vi "WPI_IMU_Loop.vi"(8 "error in":errorcluster, 11 "ADI IMU Interrupt DevRef":T1={"SimpleGyroDevRef"={"DevStatus"={"status"=FALSE, "code"=0, "source"=""}, "Handle"=0, "SPI Bus"=enum."SPI On-Board, CS0", "Device Found"=FALSE, "Sample Rate"=0.0, "Device Ready"=FALSE, "Yaw Axis"=enum."Z", "AHRS Algorithm"=enum."Complementary"}, "InterruptRef"={"DevStatus"={"status"=FALSE, "code"=0, "source"=""}, "InterruptIndex"=enum."0"}} {"SimpleGyroDevRef"."Sample Rate" min=0.25 max=100.0 step=0.25}) -> (0 "error out":errorcluster, 1 "Device Found":bool)   [LabVIEW 2015, in "FRC ADI MXP IMU.lvlib"]
doc: "Periodically reads the ADI MXP IMU valuse and makes data available for use elsewhere in your robot project. Place this block within PeriodicTasks.vi outside any loops."
uses:
  FRC ADI MXP IMU.lvlib
  WPI_AnalogDevicesIMUInterruptDevRef.ctl
  WPI_AnalogDevicesIMUDevRef.ctl
  <vilib>/Rock Robotics/SystemInterfaces/spilib/spi_bus.ctl
  <vilib>/Rock Robotics/WPI/Interrupt/WPI_InterruptRef.ctl
  <vilib>/Rock Robotics/SystemInterfaces/Interrupt/FPGA_InterruptIndex.ctl
  <vilib>/Rock Robotics/WPI/SPI/WPI_SPIDevRef.ctl
  <vilib>/Platform/TimedLoop/XDataNode/timing_clust.ctl
  <vilib>/Platform/TimedLoop/XDataNode/nitl_modes.ctl
  <vilib>/Platform/TimedLoop/XDataNode/wakeup.ctl
  <vilib>/Rock Robotics/SystemInterfaces/Interrupt/FPGA_WaitOnInterrupt.vi
  <vilib>/Rock Robotics/WPI/Utilities/WPI_UtilitiesTimebaseConstants.vi
  <vilib>/Rock Robotics/SystemInterfaces/Interrupt/FPGA_InterruptReadTimestamp.vi
  <vilib>/platform/TimedLoop/XDataNode/XDataNode.xnode
  <vilib>/ptbypt/NI_PtbyPt.lvlib
  <vilib>/Platform/TimedLoop/XDataNode/XDNodeRunTimeDep.lvlib
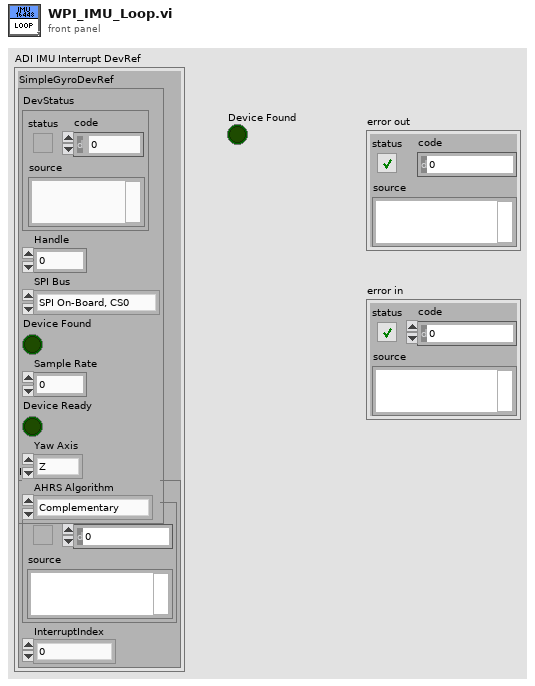
[diagram p1: front panel]
types:
  T1 = typedef "FRC ADI MXP IMU.lvlib/WPI_AnalogDevicesIMUInterruptDevRef.ctl" = cluster{"SimpleGyroDevRef":T2, "InterruptRef":T4}
  T2 = typedef "FRC ADI MXP IMU.lvlib/WPI_AnalogDevicesIMUDevRef.ctl" = cluster{"DevStatus":errorcluster, "Handle":i32, "SPI Bus":T3, "Device Found":bool, "Sample Rate":dbl, "Device Ready":bool, "Yaw Axis":enum16{"X", "Y", "Z"}, "AHRS Algorithm":enum16{"Complementary", "Madgwick"}}
  T3 = typedef "spi_bus.ctl" = enum16{"SPI On-Board, CS0", "SPI On-Board, CS1", "SPI On-Board, CS2", "SPI On-Board, CS3", "SPI MXP", "Invalid"}
  T4 = typedef "WPI_InterruptRef.ctl" = cluster{"DevStatus":errorcluster, "InterruptIndex":T5}
  T5 = typedef "FPGA_InterruptIndex.ctl" = enum8{"0", "1", "2", "3", "4", "5", "6", "7", "Invalid"}
  T6 = typedef "WPI_SPIDevRef.ctl" = cluster{"DevStatus":errorcluster, "Handle":i32, "SPI Bus":T3}
  T7 = cluster{"X Crossover":dbl, "Y Crossover":dbl, "Z Crossover":dbl, "X Range":dbl, "Y Range":dbl, "Z Range":dbl, "X Angle":dbl, "Y Angle":dbl, "Z Angle":dbl}
  T8 = cluster{"Output[0]":dbl, "Output[1]":dbl, "Output[2]":dbl}
  T9 = typedef "XDNodeRunTimeDep.lvlib/timing_clust.ctl" = cluster{"Expected End [f-1]":u64, "Actual End [f-1]":u64, "Finished Late? [f-1]":bool, "Expected End [i-1]":u64, "Actual End [i-1]":u64, "Finished Late? [i-1]":bool, "Expected Start [i]":u64, "Actual Start [i]":u64, "Expected Start [f]":u64, "Actual Start [f]":u64, "Source Name":string, "Structure Name":string, "Period":i64, "Deadline":i64, "Offset":i64, "Start":i64, "Priority":i32, "Timeout":i32, "Mode":T10, "Wakeup Reason":T11, "Error":errorcluster, "Source Type":string, "Secondary Source Type":string, "Global End Time":u64, "Global Start Time":u64, "Frame Duration":u64, "Iteration Duration":u64, "Assigned CPU":i32, "I/O Scan Engine Mode":u32}
  T10 = typedef "XDNodeRunTimeDep.lvlib/nitl_modes.ctl" = enum32{"No Change", "Process missed periods, maintain original phase", "Discard missed periods, maintain original phase", "Process missed periods, ignore original phase", "Discard missed periods, ignore original phase"}
  T11 = typedef "XDNodeRunTimeDep.lvlib/wakeup.ctl" = enum32{"Normal", "Aborted", "Asynchronous wakeup", "Timing source error", "Timed loop error", "Timeout"}
  T12 = cluster{"Data Array[0]":dbl, "Data Array[1]":dbl, "Data Array[2]":dbl, "Data Array[3]":dbl, "Data Array[4]":dbl, "Data Array[5]":dbl, "Data Array[6]":dbl, "Data Array[7]":dbl, "Data Array[8]":dbl, "Data Array[9]":dbl, "Data Array[10]":dbl}
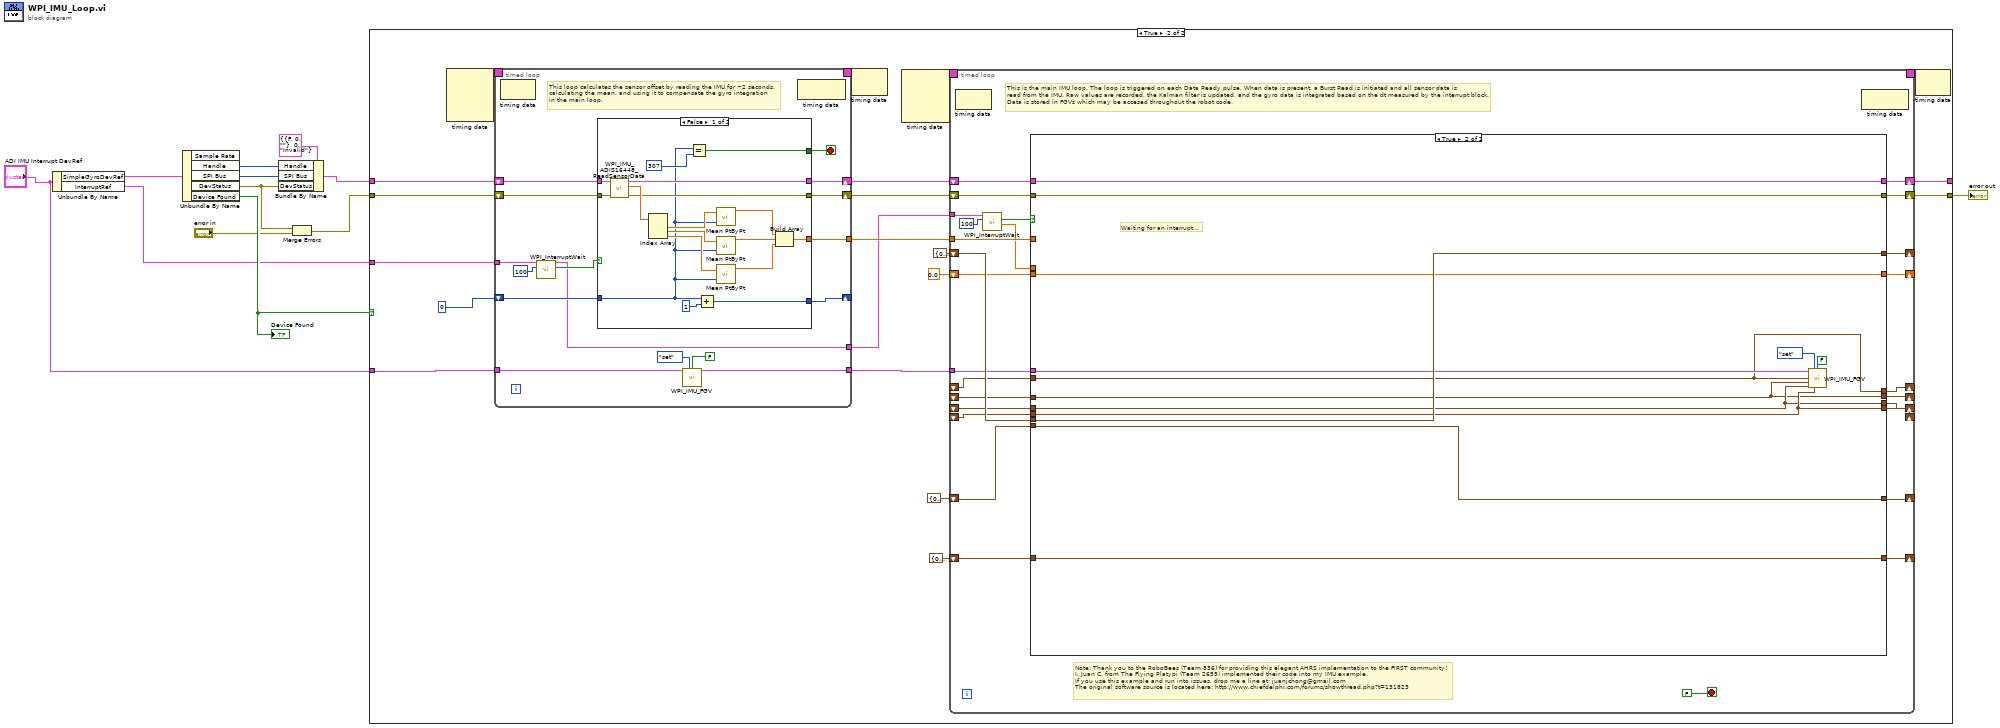
[diagram p0: block diagram]
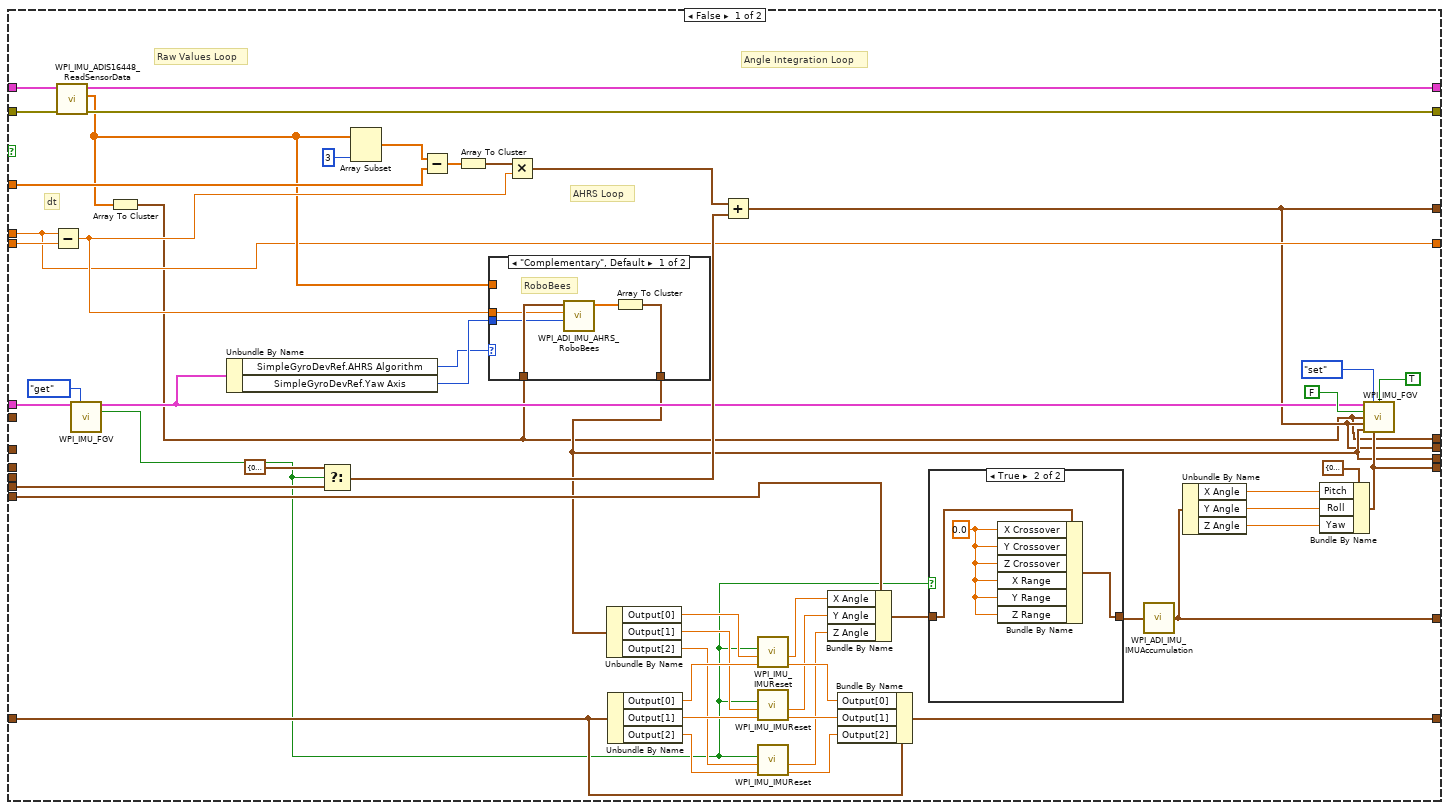
[diagram p3: hidden frame]
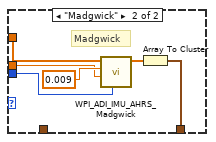
[diagram p5: hidden frame]
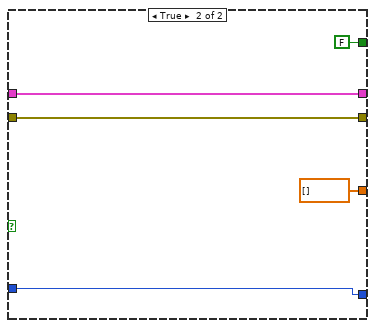
[diagram p6: hidden frame]
diagram:
  n1 = Unbundle By Name("ADI IMU Interrupt DevRef") -> ("SimpleGyroDevRef"=w6:T2, "InterruptRef"=w5:T4)
  n2 = Unbundle By Name(w6) -> ("Handle"=w11:i32, "SPI Bus"=w10:T3, "DevStatus"=w3:errorcluster, "Device Found"=w9:bool)  [unwired: 1 out]
  "Device Found" <- w9
  n3 = Bundle By Name(cluster=T6 {"DevStatus"={"status"=FALSE, "code"=0, "source"=""}, "Handle"=0, "SPI Bus"=enum."Invalid"} ("SPIDevRef out"), "Handle"=w11, "SPI Bus"=w10, "DevStatus"=w3) -> (w8:T6)
  n4 = Merge Errors(w3, "error in") -> (w1:errorcluster)
  n5 = case shown="True" w9 {
    tunnel: w8 -> [w14 w32]
    tunnel: w1 -> [w13 w31]
    tunnel: [w13 w34] -> w7
    tunnel: [w14 w33] -> _
    tunnel: "ADI IMU Interrupt DevRef" -> [_ w19]
    tunnel: w5 -> [_ w21]
    frame False {
    }
    frame True {
      n6 = node-c288() -> (w23:T9)  [unwired: 4 in]
      n7 = timed-loop {
        tunnel: [w158] -> w27
        shift-right: [w160] -> w29
        shift-left: w32 -> [w152]
        shift-right: [w161] -> w30
        shift-left: w31 -> [w151]
        shift-right: [w156] -> _
        shift-left: 0 -> [w157]
        tunnel: w21 -> [w155]
        tunnel: [w150] -> w25
        timing: w23 -> [_]
        timing-out: [_] -> w22
        tunnel: w19 -> [w148]
        tunnel: [w149] -> w16
        stop <- w159 stop-if-true
        # "This loop calculates the sensor offset by reading the IMU for ~2 seconds, \ncalculating the mean, and using it to compensate the gyro integration\nin the main loop."
        n8 = node-c288() -> ()  [unwired: 1 in, 1 out]
        n9 = call <vilib>:"WPI_InterruptWait.vi"("Timeout (ms)"=100, "InterruptRef"=w155) -> ("Timed Out"=w153:bool, "InterruptRef"=w150:T4)  [unwired: 5 in, 3 out]
        n10 = case shown="False" w153 {
          tunnel: [w179 w182] -> w161
          tunnel: [w178 w183] -> w160
          tunnel: [w173 FALSE] -> w159
          tunnel: [w169 dbl[] []] -> w158
          tunnel: w151 -> [w168 w182]
          tunnel: w152 -> [w167 w183]
          tunnel: w157 -> [w164 w185]
          tunnel: [w166 w185] -> w156
          frame False {
            n11 = call "WPI_IMU_ADIS16448_ReadSensorData.vi"("error in (no error)"=w168, "SPIDevRef in"=w167) -> ("error out"=w179:errorcluster, "Data Array"=w180:dbl[], "SPIDevRef out"=w178:T6)  [unwired: 7 in]
            n12 = Index Array(array=w180) -> (element #1=w177:dbl, element #2=w176:dbl, element #3=w175:dbl)  [unwired: 3 in]
            n13 = Equal?(x=w164, y=307) -> (x = y?=w173:bool)
            n14 = Add(x=w164, y=1) -> (x+y=w166:i32)
            n15 = call <vilib>:"Mean PtByPt.vi"("x"=w177, "sample length"=w164) -> ("mean"=w172:dbl)  [unwired: 2 in, 1 out]
            n16 = call <vilib>:"Mean PtByPt.vi"("x"=w176, "sample length"=w164) -> ("mean"=w171:dbl)  [unwired: 2 in, 1 out]
            n17 = call <vilib>:"Mean PtByPt.vi"("x"=w175, "sample length"=w164) -> ("mean"=w170:dbl)  [unwired: 2 in, 1 out]
            n18 = Build Array(w172, w171, w170) -> (w169:dbl[])
          }
          frame True {
          }
        }
        n19 = call "WPI_IMU_FGV.vi"("ADI IMU Interrupt DevRef"=w148, "Operation"=enum16{"set", "get"}."set", "Sensor Ready?"=FALSE) -> ("ADI IMU Interrupt DevRef Out"=w149:T1)  [unwired: 6 in, 6 out]
        n20 = node-c288() -> ()  [unwired: 1 in, 1 out]
      }
      n21 = node-c288(w22) -> ()  [unwired: 1 out]
      n22 = node-c288() -> (w18:T9)  [unwired: 4 in]
      n23 = timed-loop {
        shift-right: [w61] -> w33
        shift-left: w29 -> [w55]
        shift-right: [w60] -> w34
        shift-left: w30 -> [w54]
        shift-right: [w58] -> _
        shift-left: cluster{dbl, dbl, dbl} {0.0, 0.0, 0.0} -> [w57]
        tunnel: w27 -> [w56]
        tunnel: w25 -> [w52]
        shift-right: [w45] -> _
        shift-left: 0.0 ("TimeStamp") -> [w50]
        shift-right: [w47] -> _
        shift-left: T8 {"Output[0]"=0.0, "Output[1]"=0.0, "Output[2]"=0.0} -> [w49]
        tunnel: w16 -> [w46]
        timing: w18 -> [_]
        timing-out: [_] -> w17
        shift-right: [w44] -> _
        shift-left: T7 {"X Crossover"=0.0, "Y Crossover"=0.0, "Z Crossover"=0.0, "X Range"=0.0, "Y Range"=0.0, "Z Range"=0.0, "X Angle"=0.0, "Y Angle"=0.0, "Z Angle"=0.0} ("Input Data") -> [w43]
        shift-right: [w42] -> _
        shift-left: _ -> [w35]
        shift-right: [w41] -> _
        shift-left: _ -> [w36]
        shift-right: [w40] -> _
        shift-left: _ -> [w37]
        shift-right: [w39] -> _
        shift-left: _ -> [w38]
        stop <- FALSE stop-if-true
        # "Note: Thank you to the RoboBees (Team 836) for providing this elegant AHRS implementation to the FIRST community!\nI, Juan C. from The Flying Platypi (Team 2655) implemented their code into my IMU example.\nIf you use this example and run into issues, drop me a line at: juanjchong@gmail.com\nThe original software source is located here: http://www.chiefdelphi.com/forums/showthread.php?t=131823"
        # "This is the main IMU loop. The loop is triggered on each Data Ready pulse. When data is present, a Burst Read is initiated and all sensor data is \nread from the IMU. Raw values are recorded, the Kalman filter is updated, and the gyro data is integrated based on the dt measured by the interrupt block.\nData is stored in FGVs which may be accesed throughout the robot code."
        n24 = node-c288() -> ()  [unwired: 1 in, 1 out]
        n25 = call <vilib>:"WPI_InterruptWait.vi"("Timeout (ms)"=100, "InterruptRef"=w52) -> ("TimeStamp"=w51:dbl, "Timed Out"=w48:bool)  [unwired: 5 in, 3 out]
        n26 = case shown="True" w48 {
          tunnel: w55 -> [w115 w143]
          tunnel: w54 -> [w114 w142]
          tunnel: [w113 w143] -> w61
          tunnel: [w112 w142] -> w60
          tunnel: w46 -> [w98 w135]
          tunnel: [w65 w141] -> w58
          tunnel: w57 -> [w108 w141]
          tunnel: w56 -> [w104 _]
          tunnel: w51 -> [w91 _]
          tunnel: w50 -> [w100 w139]
          tunnel: w49 -> [w81 w140]
          tunnel: [w79 w140] -> w47
          tunnel: [w91 w139] -> w45
          tunnel: [w71 w138] -> w44
          tunnel: w43 -> [w80 w138]
          tunnel: [w67 w134] -> w42
          tunnel: [w66 w133] -> w41
          tunnel: [w65 w132] -> w40
          tunnel: [w64 w131] -> w39
          tunnel: w38 -> [_ w131]
          tunnel: w37 -> [_ w132]
          tunnel: w36 -> [_ w133]
          tunnel: w35 -> [_ w134]
          frame False {
            # "dt"
            # "Angle Integration Loop"
            # "AHRS Loop"
            # "Raw Values Loop"
            n27 = Subtract(x=w91, y=w100) -> (x-y=w95:dbl)
            n28 = call "WPI_IMU_ADIS16448_ReadSensorData.vi"("error in (no error)"=w114, "SPIDevRef in"=w115) -> ("error out"=w112:errorcluster, "Data Array"=w93:dbl[], "SPIDevRef out"=w113:T6)  [unwired: 7 in]
            n29 = call "WPI_IMU_FGV.vi"("ADI IMU Interrupt DevRef"=w98, "Operation"=enum16{"set", "get"}."get") -> ("ADI IMU Interrupt DevRef Out"=w96:T1, "Reset Out"=w73:bool)  [unwired: 7 in, 5 out]
            n30 = Array To Cluster(array=w93) -> (cluster=w64:T12)
            n31 = Unbundle By Name(w96) -> ("SimpleGyroDevRef.AHRS Algorithm"=w92:enum16{"Complementary", "Madgwick"}, "SimpleGyroDevRef.Yaw Axis"=w94:enum16{"X", "Y", "Z"})
            n32 = Select(t=T8 {"Output[0]"=0.0, "Output[1]"=0.0, "Output[2]"=0.0} ("cluster"), s=w73, f=w108) -> (s? t:f=w107:T8)
            n33 = Array Subset(array=w93, length=3) -> (w105:dbl[])  [unwired: 1 in]
            n34 = Subtract(x=w105, y=w104) -> (x-y=w103:dbl[])
            n35 = Array To Cluster(array=w103) -> (cluster=w102:cluster{"[0]":dbl, "[1]":dbl, "[2]":dbl})
            n36 = case shown="\"Complementary\", Default" w92 {
              tunnel: [w123 w128] -> w66
              tunnel: w64 -> [w122 _]
              tunnel: w95 -> [w121 w127]
              tunnel: w94 -> [w120 w125]
              tunnel: w93 -> [_ w126]
              frame "Complementary", Default {
                # "RoboBees"
                n37 = call "WPI_ADI_IMU_AHRS_RoboBees.vi"("Yaw Axis"=w120, "dt (s)"=w121, "IMU Rates"=w122) -> ("Output"=w124:dbl[])  [unwired: 4 in, 3 out]
                n38 = Array To Cluster(array=w124) -> (cluster=w123:T8)
              }
              frame "Madgwick" {
                # "Madgwick"
                n39 = call "WPI_ADI_IMU_AHRS_Madgwick.vi"("Yaw Axis"=w125, "dt (s)"=w127, "Beta"=0.009, "Data"=w126) -> ("Output"=w129:dbl[])  [unwired: 7 in]
                n40 = Array To Cluster(array=w129) -> (cluster=w128:T8)
              }
            }
            n41 = Multiply(x=w102, y=w95) -> (x*y=w101:cluster{"[0]":dbl, "[1]":dbl, "[2]":dbl})
            n42 = Unbundle By Name(w66) -> ("Output[0]"=w87:dbl, "Output[1]"=w86:dbl, "Output[2]"=w85:dbl)
            n43 = Unbundle By Name(w81) -> ("Output[0]"=w90:dbl, "Output[1]"=w89:dbl, "Output[2]"=w88:dbl)
            n44 = Add(x=w101, y=w107) -> (x+y=w65:cluster{dbl, dbl, dbl})
            n45 = call "WPI_IMU_IMUReset.vi"("AHRS Reset In"=w90, "Absolute Angle"=w87, "Reset"=w73) -> ("AHRS Reset Out"=w84:dbl, "Converted Output"=w78:dbl)  [unwired: 5 in]
            n46 = call "WPI_IMU_IMUReset.vi"("AHRS Reset In"=w89, "Absolute Angle"=w86, "Reset"=w73) -> ("AHRS Reset Out"=w83:dbl, "Converted Output"=w77:dbl)  [unwired: 5 in]
            n47 = call "WPI_IMU_IMUReset.vi"("AHRS Reset In"=w88, "Absolute Angle"=w85, "Reset"=w73) -> ("AHRS Reset Out"=w82:dbl, "Converted Output"=w76:dbl)  [unwired: 5 in]
            n48 = Bundle By Name(cluster=w80, "X Angle"=w78, "Y Angle"=w77, "Z Angle"=w76) -> (w74:T7)
            n49 = Bundle By Name(cluster=w81, "Output[0]"=w84, "Output[1]"=w83, "Output[2]"=w82) -> (w79:T8)
            n50 = case shown="True" w73 {
              tunnel: [w116 w118] -> w75
              tunnel: w74 -> [w116 w119]
              frame False {
              }
              frame True {
                w117 = 0.0
                n51 = Bundle By Name(cluster=w119, "X Crossover"=w117, "Y Crossover"=w117, "Z Crossover"=w117, "X Range"=w117, "Y Range"=w117, "Z Range"=w117) -> (w118:T7)
              }
            }
            n52 = call "WPI_ADI_IMU_IMUAccumulation.vi"("Input Data"=w75) -> ("Output Data"=w71:T7)
            n53 = Unbundle By Name(w71) -> ("X Angle"=w70:dbl, "Y Angle"=w69:dbl, "Z Angle"=w68:dbl)
            n54 = Bundle By Name(cluster=cluster{"Pitch":dbl, "Roll":dbl, "Yaw":dbl} {"Pitch"=0.0, "Roll"=0.0, "Yaw"=0.0} ("IMU AHRS DELTA"), "Pitch"=w70, "Roll"=w69, "Yaw"=w68) -> (w67:cluster{"Pitch":dbl, "Roll":dbl, "Yaw":dbl})
            n55 = call "WPI_IMU_FGV.vi"("ADI IMU Interrupt DevRef"=w96, "Operation"=enum16{"set", "get"}."set", "Sensor Ready?"=TRUE, "Reset"=FALSE ("Calibrated"), "IMU Data"=w64, "IMU Angles"=w65, "IMU AHRS"=w66, "IMU AHRS DELTA"=w67) -> ()  [unwired: 1 in, 7 out]
          }
          frame True {
            # "Waiting for an interrupt..."
            n56 = call "WPI_IMU_FGV.vi"("ADI IMU Interrupt DevRef"=w135, "Operation"=enum16{"set", "get"}."set", "Sensor Ready?"=FALSE, "IMU Data"=w131, "IMU Angles"=w132, "IMU AHRS"=w133, "IMU AHRS DELTA"=w134) -> ()  [unwired: 2 in, 7 out]
          }
        }
        n57 = node-c288() -> ()  [unwired: 1 in, 1 out]
      }
      n58 = node-c288(w17) -> ()  [unwired: 1 out]
    }
  }
  "error out" <- w7
